vi "cRIO Read Vendor Name.vi"(8 "error in":errorcluster, 11 "Refnum in":refnum<k20>) -> (0 "error out":errorcluster, 1 "Vendor ID":u16 format="%x", 2 "Vendor Name":string, 3 "Refnum out":refnum<k20>)   [LabVIEW 2015]
uses:
  Module/Module.lvclass
panel:
  out "Vendor Code":string
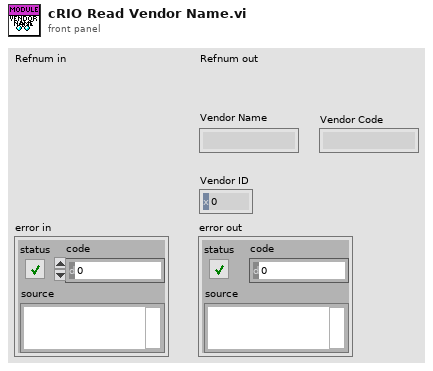
[diagram p1: front panel]
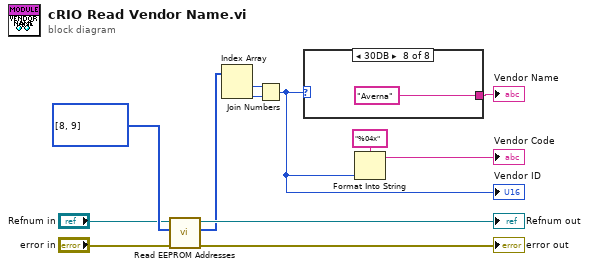
[diagram p0: block diagram]
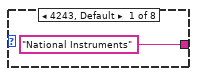
[diagram p2: hidden frame]
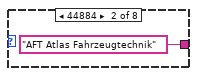
[diagram p3: hidden frame]
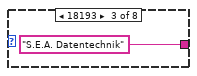
[diagram p4: hidden frame]
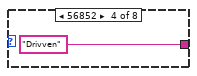
[diagram p5: hidden frame]
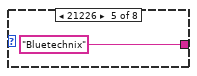
[diagram p6: hidden frame]
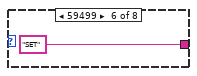
[diagram p7: hidden frame]
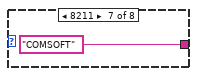
[diagram p8: hidden frame]
diagram:
  n1 = call "Read EEPROM Addresses.vi"("error in (no error)"="error in", "Addresses"=u16[] [8, 9], "Refnum in"="Refnum in") -> ("error out"=→"error out":errorcluster, "Data"=w5:u8[], "Refnum out"=→"Refnum out":refnum<k20>)  [unwired: 6 in]
  n2 = Index Array(array=w5) -> (element #1=w7:u8, element #2=w6:u8)  [unwired: 2 in]
  n3 = Join Numbers(hi=w7, lo=w6) -> ((hi.lo)=w2:u16)
  "Vendor ID" <- w2
  n4 = case shown="30DB" w2 {
    tunnel: ["National Instruments" "AFT Atlas Fahrzeugtechnik" "S.E.A. Datentechnik" "Drivven" "Bluetechnix" "SET" "COMSOFT" "Averna"] -> w4
    frame 4243, Default {
    }
    frame 44884 {
    }
    frame 18193 {
    }
    frame 56852 {
    }
    frame 21226 {
    }
    frame 59499 {
    }
    frame 8211 {
    }
    frame 12507 {
    }
  }
  "Vendor Name" <- w4
  n5 = Format Into String(format string="%04x", w2) -> (resulting string=→"Vendor Code":string)  [unwired: 2 in, 1 out]
